vi "Process components.vi"(0 "Database Entry in":refnum<class "Database Entry.lvclass">, 11 "error in (no error)":errorcluster) -> (1 "Status":string, 2 "Feet check":bool, 3 "PUT Settings":T1(array[cluster]), 4 "Database Entry out":refnum<class "Database Entry.lvclass">, 6 "Module?":bool, 8 "Aborted":bool, 10 "Assembly Settings":T1(array[cluster]), 12 "Assembly Type":string[](array[string]), 13 "Stack names":string[](array[string]), 14 "Component Settings":T1(array[cluster]), 15 "error out":errorcluster)   [LabVIEW 2021, in "Database Entry.lvclass"]
uses:
  Database Entry.lvclass
  Database Entry.lvclass/Database Entry.ctl
  Components/Stack/Stack.lvclass
panel:
  out "Selected postitions":dbl[](array[numeric])
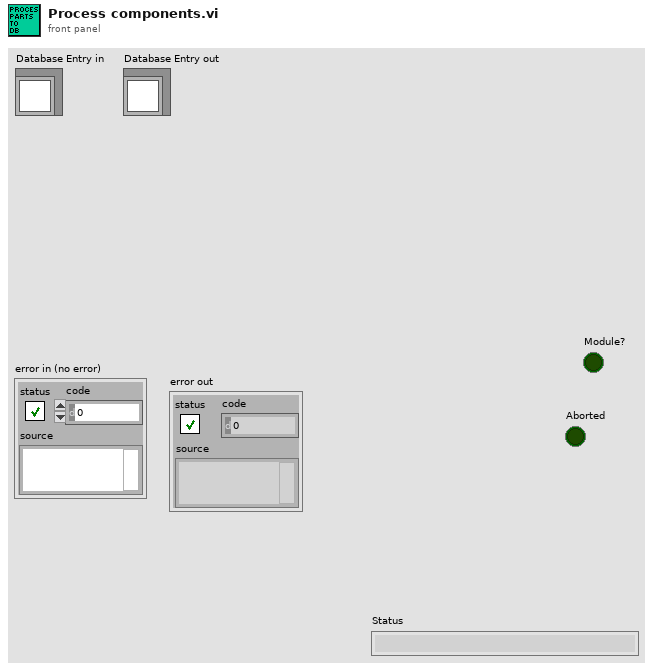
[diagram p1: front panel]
types:
  T1 = cluster{"Fixture ID":dbl, "Position":dbl, "Thickness":dbl}[]
  T2 = cluster{"Fixture ID":dbl, "Position":dbl, "Thickness":dbl}
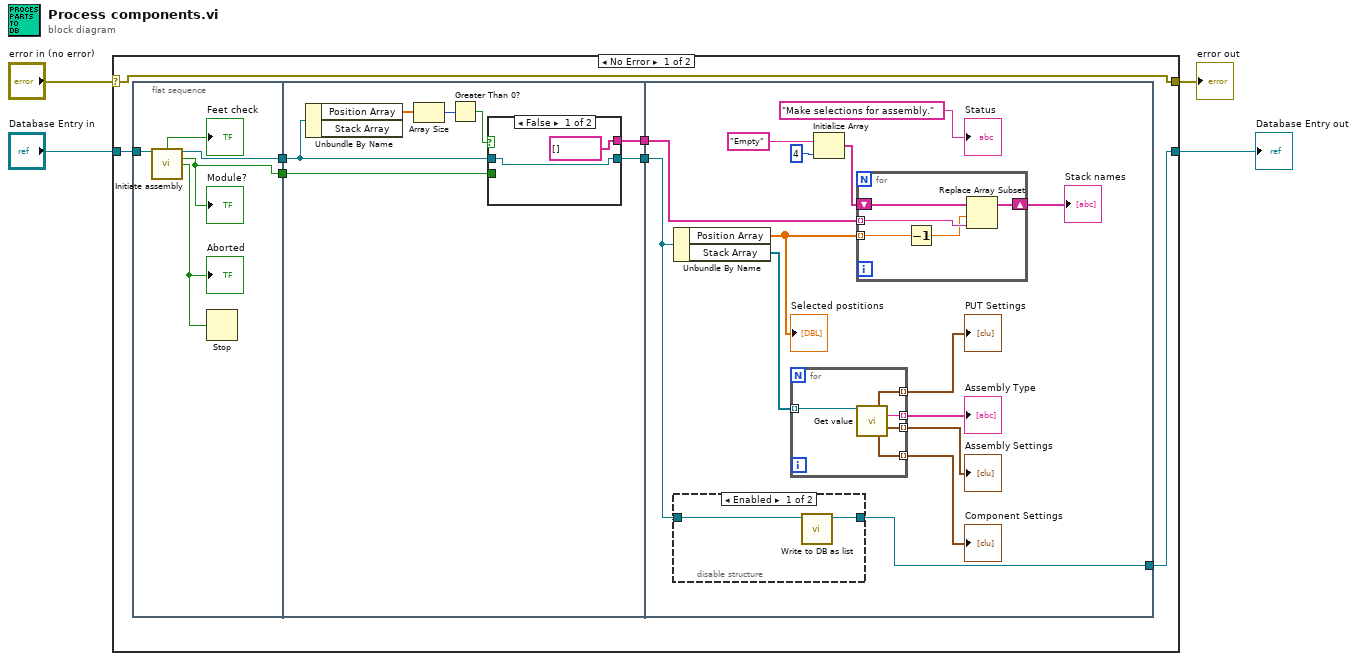
[diagram p0: block diagram]
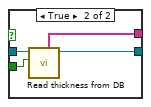
[diagram p2: hidden frame]
diagram:
  n1 = case shown="No Error" "error in (no error)" {
    selector: "error in (no error)" -> [w11 w58]
    tunnel: [w11 w58] -> w3
    tunnel: [w9 w57] -> w1
    tunnel: "Database Entry in" -> [w10 w57]
    frame No Error {
      n2 = flat-sequence {
        tunnel: w10 -> [w16]
        tunnel: [w15] -> w8
        tunnel: [w12] -> w6
        tunnel: w8 -> [w21]
        tunnel: [w23] -> w7
        tunnel: w6 -> [w22]
        tunnel: [w17] -> w5
        tunnel: w7 -> [w38]
        tunnel: [w36] -> w9
        tunnel: w5 -> [w30]
        frame #0 {
          n3 = call "Initiate assembly.vi"("Database Entry in"=w16) -> ("Feet check"=→"Feet check":bool, "Database Entry out"=w15:refnum<class "Database Entry.lvclass">, "Module?"=w12:bool, "Abort out"=w13:bool)  [unwired: 10 in, 1 out]
          "Module?" <- w12
          "Aborted" <- w13
          n4 = Stop(stop? (T)=w13) -> ()
        }
        frame #1 {
          n5 = Unbundle By Name(w21) -> ("Position Array"=w20:dbl[])  [unwired: 1 out]
          n6 = Array Size(array=w20) -> (size(s)=w19:i32)
          n7 = Greater Than 0?(x=w19) -> (x > 0?=w18:bool)
          n8 = case shown="False" w18 {
            tunnel: [w25 w29] -> w23
            tunnel: w22 -> [_ w28]
            tunnel: w21 -> [w25 w27]
            tunnel: [string[] [] w26] -> w17
            frame False {
            }
            frame True {
              n9 = call "Read thickness from DB.vi"("Module?"=w28, "Database Entry in"=w27) -> ("Database Entry out"=w29:refnum<class "Database Entry.lvclass">, "Stack names"=w26:string[])  [unwired: 5 in, 3 out]
            }
          }
        }
        frame #2 {
          n10 = Unbundle By Name(w38) -> ("Position Array"=w37:dbl[], "Stack Array"=w43:refnum<class "Stack.lvclass">[])
          "Selected postitions" <- w37
          n11 = disable-structure shown="Enabled" {
            disable-tunnel: w38 -> [w45 w46]
            disable-tunnel: [w44 w46] -> w36
            frame Enabled {
              n12 = call "Write to DB as list.vi"("Database Entry in"=w45) -> ("Database Entry out"=w44:refnum<class "Database Entry.lvclass">)  [unwired: 8 in, 2 out]
            }
            frame Disabled {
            }
          }
          n13 = for {
            tunnel: w43 -> [w56] mode=indexing
            tunnel: [w55] -> w42 mode=indexing
            tunnel: [w52] -> w41 mode=indexing
            tunnel: [w54] -> w40 mode=indexing
            tunnel: [w53] -> w39 mode=indexing
            n14 = call "Get value.vi"("Stack in"=w56) -> ("PUT Settings"=w55:T2, "Resolution Geometry"=w53:string, "Assembly Settings"=w54:T2, "Component Settings"=w52:T2)  [unwired: 9 in, 2 out]
          }
          "Assembly Settings" <- w40
          "Component Settings" <- w41
          "PUT Settings" <- w42
          "Assembly Type" <- w39
          n15 = Initialize Array("Empty", 4 ("dimension size")) -> (w32:string[])
          n16 = for {
            tunnel: w37 -> [w49] mode=indexing
            tunnel: w30 -> [w50] mode=indexing
            shift-right: [w47] -> w35
            shift-left: w32 -> [w51]
            n17 = Decrement(x=w49) -> (x-1=w48:dbl)
            n18 = Replace Array Subset(array=w51, new element=w50, index=w48) -> (w47:string[])
          }
          "Stack names" <- w35
          "Status" <- "Make selections for assembly." ("Status")
        }
      }
    }
    frame Error {
    }
  }
  "error out" <- w3
  "Database Entry out" <- w1
